vi "CreatePublicEvents.vi"(8 "error in (no error)":errorcluster, 11 "SMO":refnum<class "SMO.lvclass">) -> (0 "error out":errorcluster, 3 "SMO out":refnum<class "SMO.lvclass">)   [LabVIEW 2021, in "smo.lvlib" / "SMO.lvclass"]
uses:
  SMO.lvclass
  Typedefs/SMOState --Enum.ctl
  Typedefs/Reserve State--Enum.ctl
  SMO.lvclass/SMO.ctl
panel:
  # "For instructions on how to use the JKI State Machine Objects, examples and video tutorials, visit:\nhttp://jki.net/state-machine-objects/\n\nJKI State Machine Objects™\nhttp://jki.net/state-machine-objects/\nCopyright (C) 2005-2015, JKI <info@jki.net>\nALL RIGHTS RESERVED"
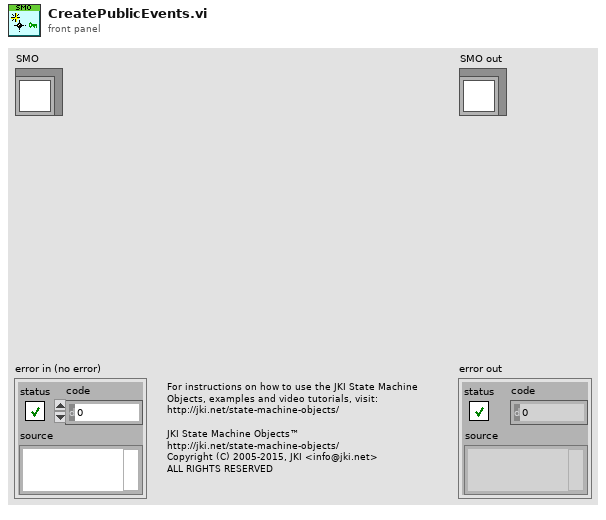
[diagram p1: front panel]
types:
  T1 = typedef "smo.lvlib/SMO.lvclass/Reserve State--Enum.ctl" = enum16{"Unreserved", "Reserved", "Self-locked"}
  T2 = typedef "smo.lvlib/SMO.lvclass/SMOState --Enum.ctl" = enum16{"unknown", "Created", "Started", "Stopped"}
  T3 = cluster{"error":refnum<user-event>, "SMO State":refnum<user-event>, "Reserve State":refnum<user-event>}
  T4 = typedef "smo.lvlib/SMO.lvclass/PrivateData--Ref.ctl" = refnum<data-value>
  T5 = typedef "smo.lvlib/SMO.lvclass/PrivateData--Cluster.ctl" = cluster{"Parent Call":T6, "Registered Processes":T7[], "Sync Notifier":refnum<notifier>, "Process Error Notifier":refnum<notifier>, "Protected Events":T8, "Public Events":T9, "SMO State":T2, "[Attributes]":variant, "Launcher Close":refnum<notifier>, "Caller Watchdog":refnum<queue>, "Accessibility":T10, "NbStaticDependencies":u32}
  T6 = typedef "smo.lvlib/SMO.lvclass/Parent Call--Enum.ctl" = enum16{"Allows parent to run", "Does not request parent to run"}
  T7 = typedef "smo.lvlib/SMO.lvclass/RegisteredProcessData--Cluster.ctl" = cluster{"Name":string, "Static VI Ref":refnum<vi>, "Running":bool, "NotifierRef":u32}
  T8 = typedef "smo.lvlib/SMO.lvclass/Protected Events.ctl" = cluster{"StopProcesses":refnum<user-event>, "AbortProcesses":refnum<user-event>, "Config Changed":refnum<user-event>, "Dependency":refnum<user-event>}
  T9 = typedef "smo.lvlib/SMO.lvclass/Public Events.ctl" = cluster{"Error":refnum<user-event>, "State":refnum<user-event>, "Reserve State":refnum<user-event>}
  T10 = typedef "smo.lvlib/SMO.lvclass/Accessibility--Cluster.ctl" = cluster{"Lock Key":string, "Reserve State":T1}
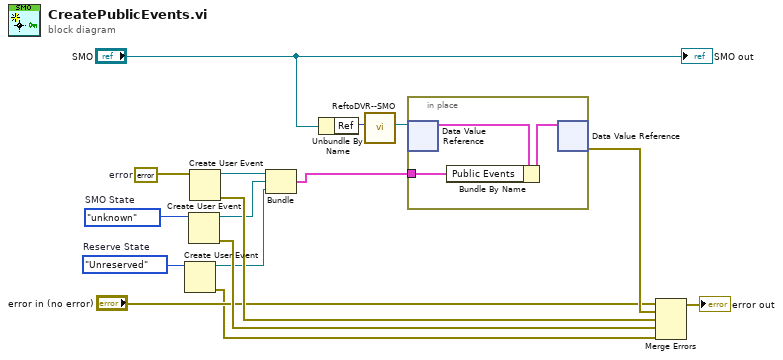
[diagram p0: block diagram]
diagram:
  w5 = Reserve_State--Enum."Unreserved"  # Reserve State
  w10 = SMOState_--Enum."unknown"  # SMO State
  w12 = errorcluster {"status"=FALSE, "code"=0, "source"=""}  # error
  n1 = Create User Event(user event datatype=w5) -> (user event=w4:refnum<user-event>, error out=w6:errorcluster)  [unwired: 1 in]
  n2 = Create User Event(user event datatype=w10) -> (user event=w9:refnum<user-event>, error out=w8:errorcluster)  [unwired: 1 in]
  n3 = Create User Event(user event datatype=w12) -> (user event=w13:refnum<user-event>, error out=w11:errorcluster)  [unwired: 1 in]
  n4 = Bundle("error"=w13, "SMO State"=w9, "Reserve State"=w4) -> (w14:T3)  [unwired: 1 in]
  n5 = Unbundle By Name("SMO") -> ("Ref"=w2:u32)
  n6 = call "ReftoDVR--SMO.vi"("Ref"=w2) -> ("Ref"=w1:T4)  [unwired: 10 in]
  n7 = in-place {
    in-place-border: w14 -> [w17]
    n8 = in-place-dvr #1(w1) -> (w19:T5)  [unwired: 1 out]
    n9 = Bundle By Name(cluster=w19, "Public Events"=w17) -> (w18:T5)
    n10 = in-place-dvr #1(w18) -> (w15:errorcluster)  [unwired: 1 out]
  }
  n11 = Merge Errors("error in (no error)", w15, w11, w8, w6) -> (→"error out":errorcluster)
  "SMO out" <- "SMO"
